vi "extract outline by gradient out.vi"(0 "input mask":u8[][](array[numeric])) -> (2 "Array out 2":u8[][](array[numeric]))   [LabVIEW 2018]
uses:
  <vilib>/vision/NI_Vision_Development_Module.lvlib
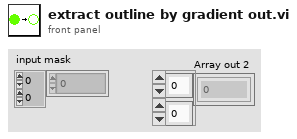
[diagram p1: front panel]
types:
  T1 = enum32{"AutoM", "Close", "Dilate", "Erode", "Gradient", "Gradient out", "Gradient in", "Hit miss", "Open", "PClose", "POpen", "Thick", "Thin"}
  T2 = typedef "IMAQ Image.ctl" = refnum<image>
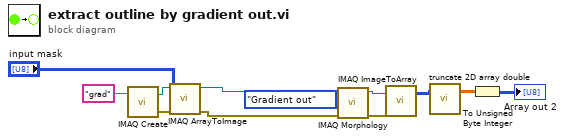
[diagram p0: block diagram]
diagram:
  n1 = call "IMAQ Create"("Image Name"="grad") -> ("New Image"=w7:T2, "error out"=w4:errorcluster)  [unwired: 4 in]
  n2 = call "IMAQ ArrayToImage"("error in (no error)"=w4, "Image Pixels (U8)"="input mask", "Image"=w7) -> ("error out"=w5:errorcluster, "Image Out"=w6:T2)  [unwired: 7 in]
  n3 = call "IMAQ Morphology"("error in (no error)"=w5, "Operation"=T1."Gradient out", "Image Src"=w6) -> ("error out"=w10:errorcluster, "Image Dst Out"=w9:T2)  [unwired: 7 in]
  n4 = call "IMAQ ImageToArray"("error in (no error)"=w10, "Image"=w9) -> ("Image Pixels (U8)"=w12:u8[][])  [unwired: 2 in, 4 out]
  n5 = call "truncate 2D array double.vi"("Array in"=w12) -> ("Array out"=w8:dbl[][])  [unwired: 2 in]
  n6 = To Unsigned Byte Integer(number=w8) -> (unsigned 8bit integer=→"Array out 2":u8[][])
